vi "Uart.vi"() -> ()   [LabVIEW 2017]
uses:
  <vilib>/myRIO/Instrument Drivers/Onboard IO/AI/typedefs/AI Reference.ctl
  <vilib>/myRIO/Common/Instrument Driver Framework/Utilities/typedefs/myRIO Generic Hardware Reference.ctl
  <vilib>/myRIO/Common/Instrument Driver Framework/Utilities/typedefs/Hardware Version Enum.ctl
  <vilib>/myRIO/Common/Instrument Driver Framework/Utilities/typedefs/myRIO v1.0 Reference.ctl
  <vilib>/myRIO/Common/Instrument Driver Framework/Utilities/typedefs/Generic FPGA Reference.ctl
  <vilib>/myRIO/Common/Instrument Driver Framework/myRIO v1.0/AI/typedefs/AI Channels List.ctl
  <vilib>/myRIO/Common/Instrument Driver Framework/myRIO v1.0/AI/typedefs/AI Channels Enum.ctl
  <vilib>/myRIO/Common/Instrument Driver Framework/Utilities/typedefs/Analog Scaling Constants List.ctl
  <vilib>/myRIO/Common/Instrument Driver Framework/Utilities/typedefs/Analog Scaling Constants.ctl
  <vilib>/userdefined/High Color/nirio_resource_hc.ctl
  <vilib>/myRIO/Instrument Drivers/Onboard IO/PWM/typedefs/PWM Reference.ctl
  <vilib>/myRIO/Common/Instrument Driver Framework/myRIO v1.0/PWM/typedefs/PWM Channels Enum.ctl
  <vilib>/myRIO/Instrument Drivers/Onboard IO/PWM/typedefs/PWM Configuration.ctl
  <vilib>/myRIO/Instrument Drivers/Onboard IO/DIO/typedefs/DIO Reference.ctl
  <vilib>/myRIO/Common/Instrument Driver Framework/myRIO v1.0/DIO/typedefs/DIO Channels List.ctl
  <vilib>/myRIO/Common/Instrument Driver Framework/myRIO v1.0/DIO/typedefs/DIO Channels Enum.ctl
  <vilib>/myRIO/Instrument Drivers/Onboard IO/UART/typedef/VISA Configuration.ctl
  <vilib>/myRIO/Common/Instrument Driver Framework/Utilities/vis/Is FPGA Ref Available.vi
  <vilib>/myRIO/Common/Instrument Driver Framework/myRIO v1.0/DIO/vis/myRIO v1.1 Open DIO.vi
  <vilib>/myRIO/Instrument Drivers/Onboard IO/DIO/vis/Write.vi
  <vilib>/myRIO/Common/Instrument Driver Framework/myRIO v1.0/PWM/vis/myRIO v1.1 Open PWM.vi
  <vilib>/myRIO/Instrument Drivers/Onboard IO/PWM/vis/Set Duty Cycle and Frequency.vi
  <vilib>/myRIO/Common/Instrument Driver Framework/myRIO v1.0/AI/vis/myRIO v1.1 Open AI.vi
  <vilib>/myRIO/Instrument Drivers/Onboard IO/AI/vis/Read.vi
  <vilib>/myRIO/Instrument Drivers/Onboard IO/DIO/vis/Read.vi
  <vilib>/myRIO/Common/Instrument Driver Framework/Utilities/vis/Validate Channels.vi
  <vilib>/myRIO/Common/Instrument Driver Framework/myRIO v1.0/DIO/vis/myRIO v1.0 Reserve DIO.vi
  <vilib>/myRIO/Common/Instrument Driver Framework/myRIO v1.0/PWM/vis/myRIO v1.0 Reserve PWM.vi
  <vilib>/myRIO/Common/Instrument Driver Framework/myRIO v1.0/AI/vis/myRIO v1.0 Reserve AI.vi
  <vilib>/myRIO/Common/Instrument Driver Framework/myRIO v1.0/Resource Manager/vis/myRIO v1.0 Reserve Channel List.vi
  <vilib>/myRIO/Common/Instrument Driver Framework/myRIO v1.0/DIO/vis/myRIO v1.0 Build MUX Configuration DIO.vi
  <vilib>/myRIO/Common/Instrument Driver Framework/myRIO v1.0/PWM/vis/myRIO v1.0 Build MUX Configuration PWM.vi
  <vilib>/myRIO/Common/Instrument Driver Framework/myRIO v1.0/AI/vis/myRIO v1.0 Build MUX Configuration AI.vi
  <vilib>/myRIO/Common/Instrument Driver Framework/myRIO v1.0/Resource Manager/vis/myRIO v1.0 Reserve Channel.vi
  <vilib>/myRIO/Common/Instrument Driver Framework/myRIO v1.0/Resource Manager/vis/myRIO v1.0 Unreserve Channel.vi
  <vilib>/myRIO/Common/Instrument Driver Framework/myRIO v1.0/Resource Manager/vis/myRIO v1.0 Create Configuration List.vi
  <vilib>/myRIO/Common/Instrument Driver Framework/myRIO v1.0/Resource Manager/vis/myRIO v1.0 Build Mutex Name.vi
  <vilib>/Utility/VariantDataType/GetNumericInfo.vi
  <vilib>/Utility/error.llb/Error Cluster From Error Code.vi
  <vilib>/myRIO/Common/Instrument Driver Framework/myRIO v1.0/myRIO v1.1 Open.vi
  <vilib>/myRIO/Common/Instrument Driver Framework/myRIO v1.0/AI/vis/myRIO v1.0 Get Scaling Constants AI.vi
  <vilib>/myRIO/Common/Instrument Driver Framework/Utilities/vis/IO Manager.vi
  <vilib>/myRIO/Common/Instrument Driver Framework/Utilities/vis/Configuration Manager.vi
  <vilib>/myRIO/Common/Instrument Driver Framework/myRIO v1.0/myRIO v1.0 Close.vi
  <vilib>/myRIO/Common/Instrument Driver Framework/myRIO v1.0/AI/vis/myRIO v1.0 Read AI.vi
  <vilib>/myRIO/Common/Instrument Driver Framework/myRIO v1.0/Resource Manager/vis/myRIO v1.0 Configure IO.vi
  <vilib>/myRIO/Common/Instrument Driver Framework/myRIO v1.0/PWM/vis/myRIO v1.0 Write PWM.vi
  <vilib>/myRIO/Common/Instrument Driver Framework/myRIO v1.0/DIO/vis/myRIO v1.0 Read DIO.vi
  <vilib>/Instr/_visa.llb/VISA Configure Serial Port (Instr).vi
  <vilib>/myRIO/Common/Instrument Driver Framework/myRIO v1.0/DIO/vis/myRIO v1.0 Write DIO.vi
  <vilib>/myRIO/Express VI/Onboard IO/AI/AI Express VI.xnode
  <vilib>/myRIO/Instrument Drivers/Onboard IO/AI/vis/myRIO AI Open.xnode
  <vilib>/myRIO/Express VI/Onboard IO/PWM/PWM Express VI.xnode
  <vilib>/myRIO/Instrument Drivers/Onboard IO/PWM/vis/myRIO PWM Open.xnode
  <vilib>/myRIO/Express VI/Onboard IO/DI/DI Express VI.xnode
  <vilib>/myRIO/Instrument Drivers/Onboard IO/DIO/vis/myRIO DIO Open.xnode
  <vilib>/myRIO/Express VI/Onboard IO/UART/UART Express VI.xnode
  <vilib>/myRIO/Express VI/Onboard IO/DO/DO Express VI.xnode
  <vilib>/myRIO/Instrument Drivers/Onboard IO/PWM/PWM.lvlib
  <vilib>/myRIO/Instrument Drivers/Onboard IO/UART/UART.lvlib
  <vilib>/myRIO/Instrument Drivers/Onboard IO/AI/AI.lvlib
  <vilib>/myRIO/Instrument Drivers/Onboard IO/DIO/DIO.lvlib
panel:
  in  "Gray++":bool
  in  "Pink++":bool
  in  "Black++":bool
  out "Actual Distance":i32
  in  "End Time (s)":dbl=60.0
  out "Elapsed Time":dbl
  out "LCD Bottom":string
  out "LCD Top":string
  out "Current Points":i16
  in  "Score Array":i16[](array[numeric])
  out "Solenoid 2":bool
  out "Solenoid 1":bool
  out "Black Target  (-45 to 45)":i16
  out "Pink Target (-40 to 40)":i16
  out "Gray Target (-15 to -90)":i16
  out "If Ready":bool
  out "Numeric":dbl
  out "Servo Gun Position":i32
  out "JoyStick Direction":string
  out "JoyStick Input":dbl
  out "Gun Fire Button":bool
  out "Range to Check":i32
  out "TOF Last 20 Reading":i32[](array[numeric])
  out "to LCD":string
  out "Byte Output":i32[](array[numeric])
  out "Distance(mm)":i32
  out "Byte Array of Ardunio String":i32[](array[numeric])
  out "Length of Ardunio Output":i32
  in  "Game Terminate":bool
  out "error out":errorcluster
  in  "error in (no error)":errorcluster
  out "Ardunio Output":string
  # "Target Control"
  # "Player Control Info"
  # "TOF input and output"
  # "Game Statistics"
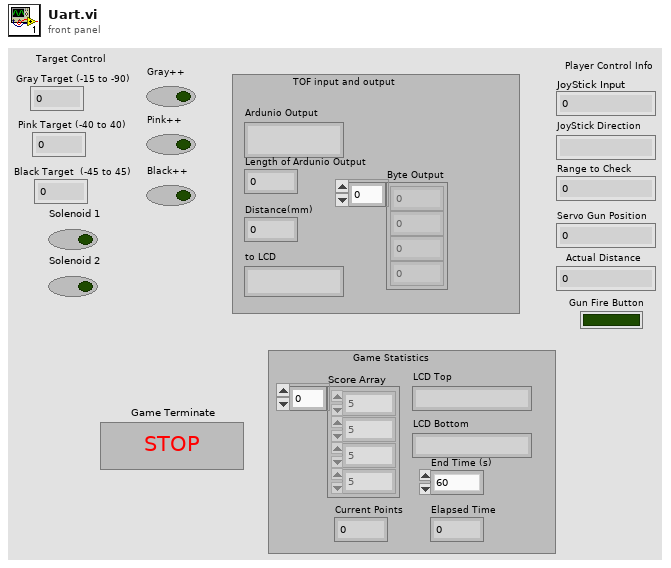
[diagram p1: front panel]
types:
  T1 = typedef "DIO.lvlib/DIO Reference.ctl" = cluster{"myRIO Reference":T2, "DIO Channels List":T6}
  T2 = typedef "myRIO Generic Hardware Reference.ctl" = cluster{"myRIO Model":T3, "myRIO Hardware Reference":T4}
  T3 = typedef "Hardware Version Enum.ctl" = enum16{"Unknown", "myRIO-1900", "myRIO-1950", "roboRIO", "NI ELVIS RIO CM"}
  T4 = typedef "myRIO v1.0 Reference.ctl" = cluster{"Generic FPGA Reference":T5, "Allow multiple opens":bool}
  T5 = typedef "Generic FPGA Reference.ctl" = refnum<k20>
  T6 = typedef "DIO Channels List.ctl" = T7[]
  T7 = typedef "DIO Channels Enum.ctl" = enum16{"Not Connected", "C/DIO0", "C/DIO1", "C/DIO2", "C/DIO3", "C/DIO4", "C/DIO5", "C/DIO6", "C/DIO7", "A/DIO0", "A/DIO1", "A/DIO2", "A/DIO3", "A/DIO4", "A/DIO5", "A/DIO6", "A/DIO7", "A/DIO8", "A/DIO9", "A/DIO10", "A/DIO11", "A/DIO12", "A/DIO13", "A/DIO14", "A/DIO15", "B/DIO0", "B/DIO1", "B/DIO2", "B/DIO3", "B/DIO4", "B/DIO5", "B/DIO6", "B/DIO7", "B/DIO8", "B/DIO9", "B/DIO10", "B/DIO11", "B/DIO12", "B/DIO13", "B/DIO14", "B/DIO15", "LED0", "LED1", "LED2", "LED3", "Button0", "DIO/DIO0", "DIO/DIO1", "DIO/DIO2", "DIO/DIO3", "DIO/DIO4", "DIO/DIO5", "DIO/DIO6", "DIO/DIO7", "DIO/DIO8", "DIO/DIO9", "SPI/CS0", "SPI/CS1", "SPI/CS2", "SPI/CS3", "LED RADIO (Green)", "LED RADIO (Red)", "LED COMM (Green)", "LED COMM (Red)", "LED MODE (Green)", "LED MODE (Red)"}
  T8 = typedef "nirio_resource_hc.ctl" = tag
  T9 = typedef "PWM.lvlib/PWM Reference.ctl" = cluster{"myRIO Reference":T2, "PWM Channels Enum":T10, "PWM Configuration":T11}
  T10 = typedef "PWM Channels Enum.ctl" = enum16{"Not Connected", "C/PWM0", "C/PWM1", "A/PWM0", "A/PWM1", "A/PWM2", "B/PWM0", "B/PWM1", "B/PWM2", "PWM/PWM0", "PWM/PWM1", "PWM/PWM2", "PWM/PWM3", "PWM/PWM4", "PWM/PWM5", "PWM/PWM6", "PWM/PWM7", "PWM/PWM8", "PWM/PWM9"}
  T11 = typedef "PWM.lvlib/PWM Configuration.ctl" = cluster{"Frequency":dbl, "Duty Cycle":dbl}
  T12 = typedef "UART.lvlib/VISA Configuration.ctl" = cluster{"baud rate (9600)":u32, "data bits (8)":u16, "parity (0:none)":enum16{"None", "Odd", "Even", "Mark", "Space"}, "stop bits (10: 1 bit)":u16, "flow control (0:none)":u16, "termination char\n(0xA = '\\n' = LF) ":u8, "Enable Termination\nChar (T)":bool, "timeout (10sec)":u32}
  T13 = typedef "I2C.lvlib/I2C Reference.ctl" = cluster{"myRIO Reference":T2, "I2C Channels Enum":T14, "I2C Configuration":T15}
  T14 = typedef "I2C Channels Enum.ctl" = enum16{"Not Connected", "A/I2C", "B/I2C", "I2C/I2C"}
  T15 = typedef "I2C.lvlib/I2C Configuration.ctl" = cluster{"I2C Transfer Rate":T16}
  T16 = typedef "I2C.lvlib/I2C Transfer Rate.ctl" = enum16{"Standard mode (100 kbps)", "Fast mode (400 kbps)"}
  T17 = typedef "AI.lvlib/AI Reference.ctl" = cluster{"myRIO Reference":T2, "AI Channels List":T18, "AI Scaling Constants List":T20}
  T18 = typedef "AI Channels List.ctl" = T19[]
  T19 = typedef "AI Channels Enum.ctl" = enum16{"Not Connected", "AudioIn/Left", "AudioIn/Right", "C/AI0", "C/AI1", "A/AI0", "A/AI1", "A/AI2", "A/AI3", "B/AI0", "B/AI1", "B/AI2", "B/AI3", "AI/AI0", "AI/AI1", "AI/AI2", "AI/AI3"}
  T20 = typedef "Analog Scaling Constants List.ctl" = T21[]
  T21 = typedef "Analog Scaling Constants.ctl" = cluster{"LSB Weight (Volts)":dbl, "Offset (Volts)":dbl, "Signed?":bool}
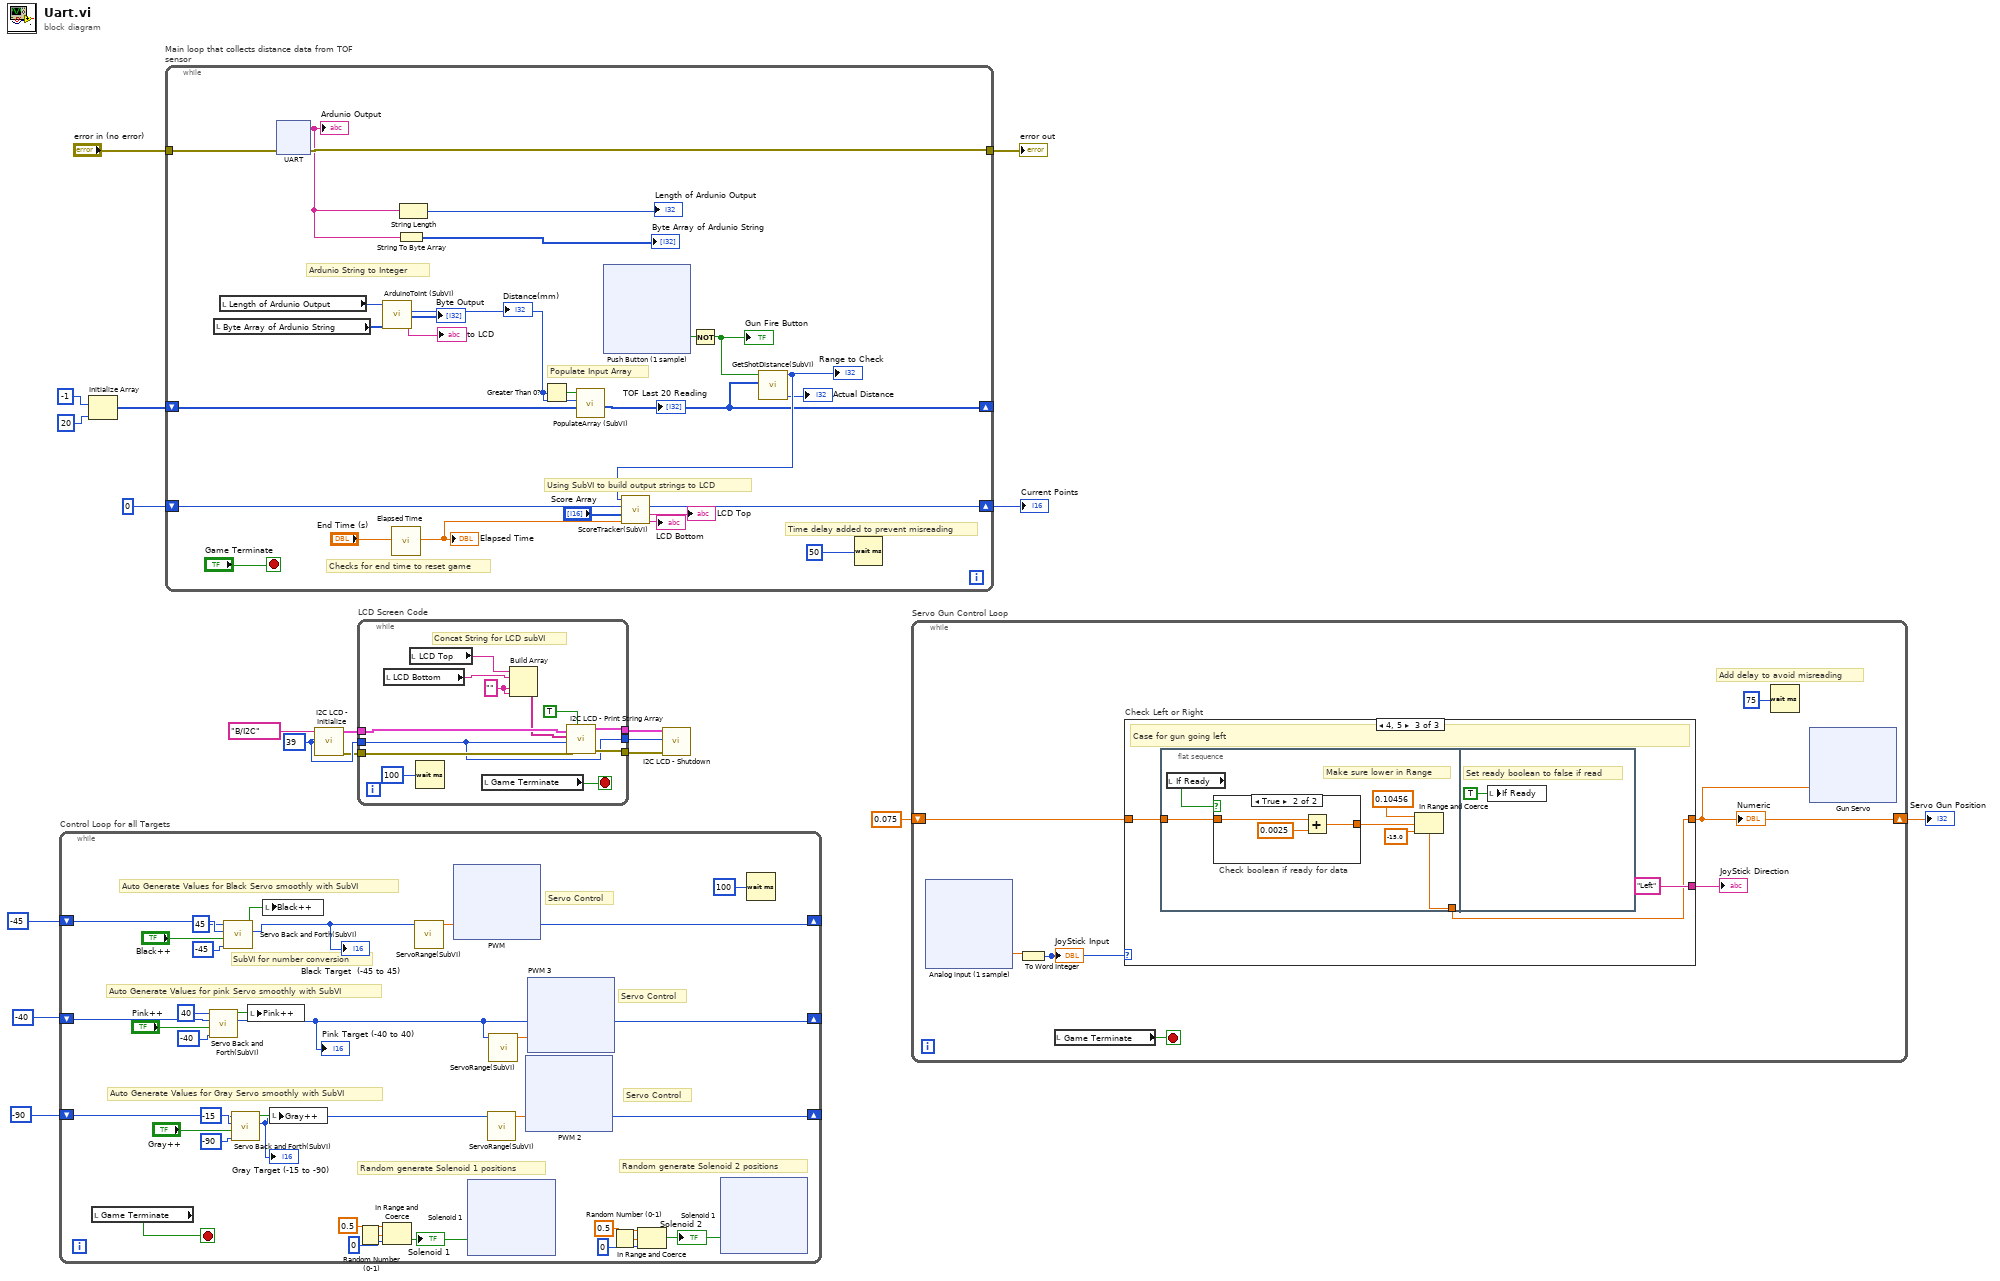
[diagram p0: block diagram]
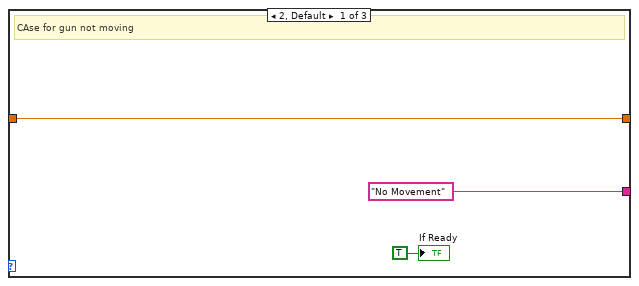
[diagram p2: hidden frame]
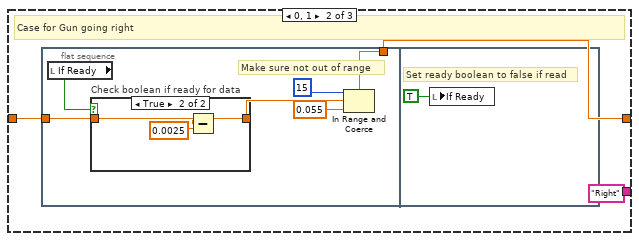
[diagram p3: hidden frame]
diagram:
  w9 = 39
  n1 = while "Control Loop for all Targets" {
    shift-right: [w41] -> _
    shift-left: -45 -> [w45]
    shift-right: [w28] -> _
    shift-left: -40 -> [w39]
    shift-right: [w29] -> _
    shift-left: -90 -> [w34]
    stop <- w46 stop-if-true
    # "Servo Control"
    # "Servo Control"
    # "Servo Control"
    # "SubVI for number conversion"
    # "Random generate Solenoid 2 positions"
    # "Random generate Solenoid 1 positions"
    # "Auto Generate Values for Black Servo smoothly with SubVI"
    # "Auto Generate Values for Gray Servo smoothly with SubVI"
    # "Auto Generate Values for pink Servo smoothly with SubVI"
    n2 = local read "Game Terminate"() -> (w46:bool)
    n3 = call "Servo Back and Forth(SubVI).vi"("Upper Bound"=40, "Original Value"=w39, "Increment in"="Pink++", "Lower Bound"=-40) -> ("Increment out"=w35:bool, "New Value"=w28:i32)  [unwired: 5 in]
    "Pink Target (-40 to 40)" <- w28
    n4 = call "Servo Back and Forth(SubVI).vi"("Upper Bound"=45, "Original Value"=w45, "Increment in"="Black++", "Lower Bound"=-45) -> ("Increment out"=w43:bool, "New Value"=w41:i32)  [unwired: 5 in]
    "Black Target  (-45 to 45)" <- w41
    n5 = call "Servo Back and Forth(SubVI).vi"("Upper Bound"=-15, "Original Value"=w34, "Increment in"="Gray++", "Lower Bound"=-90) -> ("Increment out"=w30:bool, "New Value"=w29:i32)  [unwired: 5 in]
    "Gray Target (-15 to -90)" <- w29
    n6 = local write "Pink++"(w35) -> ()
    n7 = local write "Black++"(w43) -> ()
    n8 = local write "Gray++"(w30) -> ()
    n9 = Random Number (0-1)() -> (number: 0 to 1=w27:dbl)
    n10 = In Range and Coerce(upper limit=0.5, x=w27, lower limit=0) -> (In Range?=w24:bool)  [unwired: 1 out]
    "Solenoid 1" <- w24
    n11 = call "ServoRange(SubVI).vi"("Gray Target (-15 to -90)"=w41) -> ("Numeric"=w48:dbl)  [unwired: 10 in]
    n12 = xnode "PWM"("Duty Cycle"=w48) -> ()  [unwired: 1 in, 1 out]
    n13 = xnode "Solenoid 1"("A/DIO14 (Pin 32)"=w24) -> ()  [unwired: 1 in, 1 out]
    n14 = call "ServoRange(SubVI).vi"("Gray Target (-15 to -90)"=w29) -> ("Numeric"=w49:dbl)  [unwired: 10 in]
    n15 = call "ServoRange(SubVI).vi"("Gray Target (-15 to -90)"=w28) -> ("Numeric"=w47:dbl)  [unwired: 10 in]
    n16 = xnode "PWM 2"("Duty Cycle"=w49) -> ()  [unwired: 1 in, 1 out]
    n17 = xnode "PWM 3"("Duty Cycle"=w47) -> ()  [unwired: 1 in, 1 out]
    n18 = Random Number (0-1)() -> (number: 0 to 1=w21:dbl)
    n19 = In Range and Coerce(upper limit=0.5, x=w21, lower limit=0) -> (In Range?=w20:bool)  [unwired: 1 out]
    "Solenoid 2" <- w20
    n20 = xnode "Solenoid 1"("A/DIO15 (Pin 34)"=w20) -> ()  [unwired: 1 in, 1 out]
    n21 = Wait (ms)(milliseconds to wait=100) -> ()  [unwired: 1 out]
  }
  n22 = Initialize Array(-1, 20) -> (w15:i32[])
  n23 = while "Main loop that collects distance data from TOF sensor" {
    tunnel: "error in (no error)" -> [w251]
    tunnel: [w250] -> w18
    shift-right: [w227] -> _
    shift-left: w15 -> [w239]
    shift-right: [w235] -> w11
    shift-left: 0 -> [w236]
    stop <- "Game Terminate" stop-if-true
    # "Using SubVI to build output strings to LCD"
    # "Checks for end time to reset game"
    # "Populate Input Array"
    # "Ardunio String to Integer"
    # "Time delay added to prevent misreading"
    n24 = local read "Byte Array of Ardunio String"() -> (w242:i32[])
    n25 = local read "Length of Ardunio Output"() -> (w244:i32)
    n26 = xnode "UART"("error in (no error)"=w251) -> ("error out"=w250:errorcluster, "Characters Read"=w246:string)
    "Ardunio Output" <- w246
    n27 = call "ArduinoToInt (SubVI).vi"("Byte Array of Ardunio String"=w242, "Length of Ardunio Output"=w244) -> ("String"=→"to LCD":string, "Numeric"=w238:i32, "Array"=→"Byte Output":i32[])  [unwired: 7 in]
    "Distance(mm)" <- w238
    n28 = call "Elapsed Time"("Time Target (s)"="End Time (s)") -> ("Elapsed Time (s)"=w231:dbl)  [unwired: 11 in, 7 out]
    "Elapsed Time" <- w231
    n29 = String To Byte Array(string=w246) -> (unsigned byte array=→"Byte Array of Ardunio String":u8[])
    n30 = String Length(string=w246) -> (length=→"Length of Ardunio Output":i32)
    n31 = Greater Than 0?(x=w238) -> (x > 0?=w240:bool)
    n32 = call "PopulateArray (SubVI).vi"("Array in"=w239, "Numeric"=w238, "Boolean"=w240) -> ("Array out"=w227:i32[])  [unwired: 8 in]
    "TOF Last 20 Reading" <- w227
    n33 = xnode "Push Button (1 sample)"() -> ("B/DIO9 (Pin 29)"=w228:bool)  [unwired: 1 in, 1 out]
    n34 = Not(x=w228) -> (.not. x?=w229:bool)
    "Gun Fire Button" <- w229
    n35 = call "GetShotDistance(SubVI).vi"("Array in"=w227, "Gun Fire Button"=w229) -> ("Current Dist"=→"Actual Distance":i16, "Numeric"=w237:i16)  [unwired: 8 in]
    "Range to Check" <- w237
    n36 = call "ScoreTracker(SubVI).vi"("Elapsed Time"=w231, "Score Array"="Score Array", "Numeric in"=w236, "Numeric 3"=w237) -> ("LCD Bottom"=→"LCD Bottom":string, "LCD Top"=→"LCD Top":string, "Numeric out"=w235:i32)  [unwired: 5 in]
    n37 = Wait (ms)(milliseconds to wait=50) -> ()  [unwired: 1 out]
  }
  "error out" <- w18
  "Current Points" <- w11
  n38 = call "I2C LCD - Initialize.vi"("Slave Address (7-bit)"=w9, "Channel Name"=tag "B/I2C") -> ("error out"=w4:errorcluster, "I2C Ref Out"=w7:T13)  [unwired: 8 in]
  n39 = while "LCD Screen Code" {
    tunnel: w7 -> [w314]
    tunnel: [w315] -> w8
    tunnel: w4 -> [w313]
    tunnel: [w312] -> w5
    tunnel: w9 -> [w311]
    tunnel: [w311] -> w10
    stop <- w308 stop-if-true
    w307 = ""
    # "Concat String for LCD subVI"
    n40 = local read "LCD Bottom"() -> (w304:string)
    n41 = local read "LCD Top"() -> (w305:string)
    n42 = Wait (ms)(milliseconds to wait=100) -> ()  [unwired: 1 out]
    n43 = local read "Game Terminate"() -> (w308:bool)
    n44 = Build Array(w305, w304, w307, w307) -> (w309:string[])
    n45 = call "I2C LCD - Print String Array.vi"("Back Light"=TRUE, "error in (no error)"=w313, "Slave Address (7-bit)"=w311, "String Array"=w309, "I2C Ref  in"=w314) -> ("error out"=w312:errorcluster, "I2C Ref Out"=w315:T13)  [unwired: 5 in]
  }
  n46 = call "I2C LCD - Shutdown.vi"("error in (no error)"=w5, "Slave Address (7-bit)"=w10, "I2C Ref Out"=w8) -> ()  [unwired: 8 in, 1 out]
  n47 = while "Servo Gun Control Loop" {
    shift-right: [w318] -> w13
    shift-left: 0.075 -> [w319]
    stop <- w316 stop-if-true
    # "Add delay to avoid misreading"
    n48 = xnode "Analog input (1 sample)"() -> ("Control X Input (A/AI0 (Pin 3))"=w322:dbl)  [unwired: 1 in, 1 out]
    n49 = To Word Integer(number=w322) -> (16bit integer=w321:i16)
    "JoyStick Input" <- w321
    n50 = local read "Game Terminate"() -> (w316:bool)
    n51 = case "Check Left or Right" shown="4, 5" w321 {
      tunnel: ["No Movement" "Right" "Left"] -> w320
      tunnel: [w359 w361 w375] -> w318
      tunnel: w319 -> [w359 w362 w376]
      frame 2, Default {
        # "CAse for gun not moving"
        "If Ready" <- TRUE
      }
      frame 0, 1 {
        # "Case for Gun going right"
        n52 = flat-sequence {
          tunnel: w362 -> [w369]
          tunnel: [w365] -> w361
          frame #0 {
            # "Make sure not out of range"
            n53 = local read "If Ready"() -> (w368:bool)
            n54 = case "Check boolean if ready for data" shown="True" w368 {
              tunnel: w369 -> [w370 w372]
              tunnel: [w370 w371] -> w367
              frame False {
              }
              frame True {
                n55 = Subtract(x=w372, y=0.0025) -> (x-y=w371:dbl)
              }
            }
            n56 = In Range and Coerce(upper limit=15, x=w367, lower limit=0.055) -> (coerced(x)=w365:dbl)  [unwired: 1 out]
          }
          frame #1 {
            # "Set ready boolean to false if read"
            n57 = local write "If Ready"(TRUE) -> ()
          }
        }
      }
      frame 4, 5 {
        # "Case for gun going left"
        n58 = flat-sequence {
          tunnel: w376 -> [w383]
          tunnel: [w379] -> w375
          frame #0 {
            # "Make sure lower in Range"
            n59 = local read "If Ready"() -> (w382:bool)
            n60 = case "Check boolean if ready for data" shown="True" w382 {
              tunnel: w383 -> [w384 w386]
              tunnel: [w384 w385] -> w380
              frame False {
              }
              frame True {
                n61 = Add(x=w386, y=0.0025) -> (x+y=w385:dbl)
              }
            }
            n62 = In Range and Coerce(upper limit=0.10456, x=w380, lower limit=-15.0) -> (coerced(x)=w379:dbl)  [unwired: 1 out]
          }
          frame #1 {
            # "Set ready boolean to false if read"
            n63 = local write "If Ready"(TRUE) -> ()
          }
        }
      }
    }
    "JoyStick Direction" <- w320
    "Numeric" <- w318
    n64 = Wait (ms)(milliseconds to wait=75) -> ()  [unwired: 1 out]
    n65 = xnode "Gun Servo"("Duty Cycle"=w318) -> ()  [unwired: 1 in, 1 out]
  }
  "Servo Gun Position" <- w13
